vi "Agilent 428X Series Calculated Accuracy Application.vi"(8 "error in (no error)":errorcluster, 9 "Meas. Type (0:Z,Y)":T1(ring), 10 "Temperature (5 C)":dbl=5.0 min=5.0 max=45.0 format="%.2f", 11 "VISA resource name":refnum<visa-resource-name>) -> (0 "error out":errorcluster, 1 "Relative Accuracy":dbl format="%.3f", 2 "Absolute Accuracy":dbl format="%.3f", 3 "VISA resource name out":refnum<visa-resource-name>)   [LabVIEW 2015]
doc: "This application VI is to calulate the absolute and relative accuracy of user specified type measurement, Application VI can calculate \nZ,Y,L,C R,X.G, B, D, Q, Theta, Rp, and Rs absolute and relative accuracy."
uses:
  <instrlib>/Agilent 428X Series/Agilent 428X Series.lvlib
panel:
  # "© Copyright 2005 National Instruments Corporation.  All Rights Reserved."
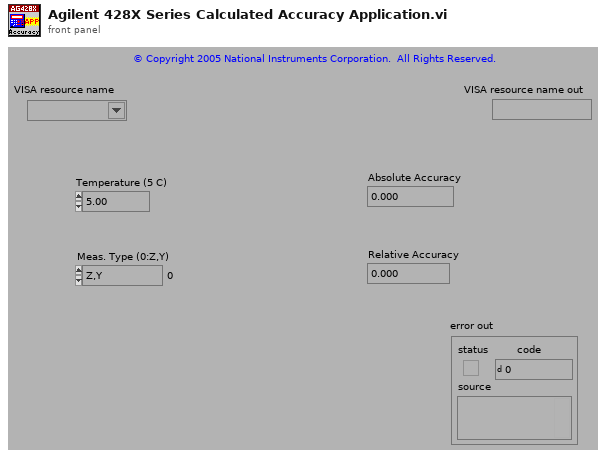
[diagram p1: front panel]
types:
  T1 = enum16{"Z,Y", "L C X B", "R G", "D", "Q", "DEGREE", "G(Cp-G Lp-G)", "Rp", "Rs"}
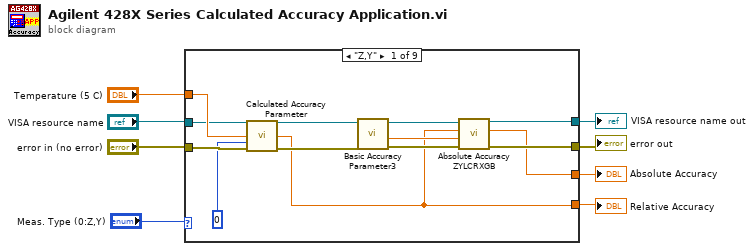
[diagram p0: block diagram]
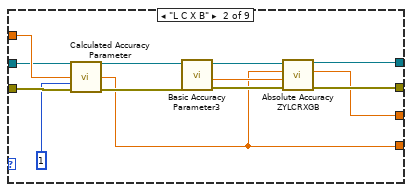
[diagram p2: hidden frame]
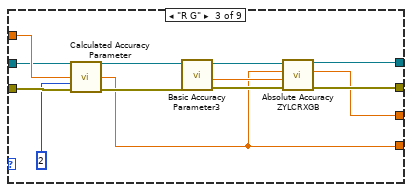
[diagram p3: hidden frame]
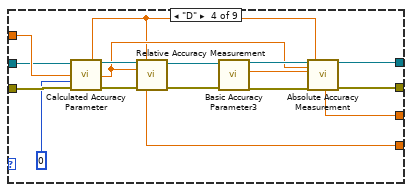
[diagram p4: hidden frame]
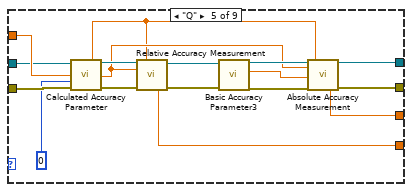
[diagram p5: hidden frame]
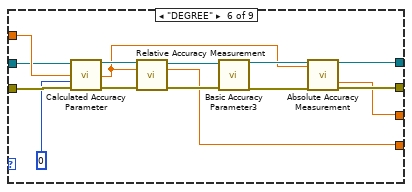
[diagram p6: hidden frame]
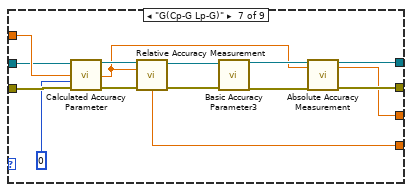
[diagram p7: hidden frame]
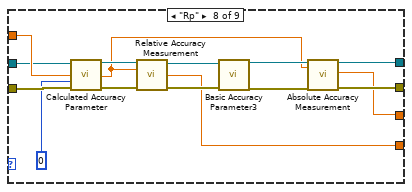
[diagram p8: hidden frame]
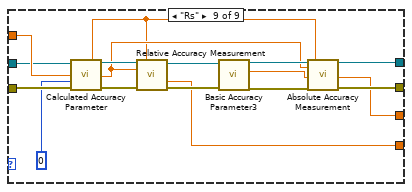
[diagram p9: hidden frame]
diagram:
  n1 = case shown="\"Z,Y\"" "Meas. Type (0:Z,Y)" {
    tunnel: "Temperature (5 C)" -> [w21 w34 w47 w64 w81 w96 w111 w126 w143]
    tunnel: "VISA resource name" -> [w20 w33 w46 w63 w80 w95 w110 w125 w142]
    tunnel: "error in (no error)" -> [w19 w32 w45 w62 w79 w94 w109 w124 w141]
    tunnel: [w13 w26 w39 w49 w68 w82 w97 w112 w127] -> w4
    tunnel: [w11 w24 w37 w58 w75 w90 w105 w120 w137] -> w3
    tunnel: [w10 w23 w36 w57 w74 w89 w104 w119 w136] -> w2
    tunnel: [w9 w22 w35 w52 w67 w84 w98 w113 w130] -> w1
    frame "Z,Y" {
      n2 = call <instrlib>:"Calculated Accuracy Parameter.vi"("VISA resource name"=w20, "Temperature (5 C)"=w21, "Meas. Type (0:Z,Y)"=0, "error in (no error)"=w19) -> ("VISA resource name out"=w18:refnum<visa-resource-name>, "Ae Accuracy"=w13:dbl, "error out"=w17:errorcluster)  [unwired: 8 in, 1 out]
      n3 = call <instrlib>:"Basic Accuracy Parameter3.vi"("error in (no error)"=w17, "VISA resource name"=w18) -> ("error out"=w16:errorcluster, "Acal"=w14:dbl, "VISA resource name out"=w15:refnum<visa-resource-name>)  [unwired: 6 in, 1 out]
      n4 = call <instrlib>:"Absolute Accuracy ZYLCRXGB.vi"("error in (no error)"=w16, "Acal"=w14, "Ae"=w13, "VISA resource name"=w15) -> ("error out"=w10:errorcluster, "Absolute Accuracy"=w9:dbl, "VISA resource name out"=w11:refnum<visa-resource-name>)  [unwired: 5 in]
    }
    frame "L C X B" {
      n5 = call <instrlib>:"Calculated Accuracy Parameter.vi"("VISA resource name"=w33, "Temperature (5 C)"=w34, "Meas. Type (0:Z,Y)"=1, "error in (no error)"=w32) -> ("VISA resource name out"=w31:refnum<visa-resource-name>, "Ae Accuracy"=w26:dbl, "error out"=w30:errorcluster)  [unwired: 8 in, 1 out]
      n6 = call <instrlib>:"Basic Accuracy Parameter3.vi"("error in (no error)"=w30, "VISA resource name"=w31) -> ("error out"=w29:errorcluster, "Acal"=w27:dbl, "VISA resource name out"=w28:refnum<visa-resource-name>)  [unwired: 6 in, 1 out]
      n7 = call <instrlib>:"Absolute Accuracy ZYLCRXGB.vi"("error in (no error)"=w29, "Acal"=w27, "Ae"=w26, "VISA resource name"=w28) -> ("error out"=w23:errorcluster, "Absolute Accuracy"=w22:dbl, "VISA resource name out"=w24:refnum<visa-resource-name>)  [unwired: 5 in]
    }
    frame "R G" {
      n8 = call <instrlib>:"Calculated Accuracy Parameter.vi"("VISA resource name"=w46, "Temperature (5 C)"=w47, "Meas. Type (0:Z,Y)"=2, "error in (no error)"=w45) -> ("VISA resource name out"=w44:refnum<visa-resource-name>, "Ae Accuracy"=w39:dbl, "error out"=w43:errorcluster)  [unwired: 8 in, 1 out]
      n9 = call <instrlib>:"Basic Accuracy Parameter3.vi"("error in (no error)"=w43, "VISA resource name"=w44) -> ("error out"=w42:errorcluster, "Acal"=w40:dbl, "VISA resource name out"=w41:refnum<visa-resource-name>)  [unwired: 6 in, 1 out]
      n10 = call <instrlib>:"Absolute Accuracy ZYLCRXGB.vi"("error in (no error)"=w42, "Acal"=w40, "Ae"=w39, "VISA resource name"=w41) -> ("error out"=w36:errorcluster, "Absolute Accuracy"=w35:dbl, "VISA resource name out"=w37:refnum<visa-resource-name>)  [unwired: 5 in]
    }
    frame "D" {
      n11 = call <instrlib>:"Calculated Accuracy Parameter.vi"("VISA resource name"=w63, "Temperature (5 C)"=w64, "Meas. Type (0:Z,Y)"=0, "error in (no error)"=w62) -> ("Frequency Used"=w48:dbl, "VISA resource name out"=w56:refnum<visa-resource-name>, "Ae Accuracy"=w51:dbl, "error out"=w55:errorcluster)  [unwired: 8 in]
      n12 = call <instrlib>:"Relative Accuracy Measurement.vi"("VISA resource name"=w56, "Frequency (20)"=w48, "Ae Accuracy (0.05)"=w51, "error in (no error)"=w55) -> ("VISA resource name out"=w54:refnum<visa-resource-name>, "D Accuracy"=w49:dbl, "error out"=w53:errorcluster)  [unwired: 4 in, 5 out]
      n13 = call <instrlib>:"Basic Accuracy Parameter3.vi"("error in (no error)"=w53, "VISA resource name"=w54) -> ("error out"=w61:errorcluster, "Radcal"=w50:dbl, "VISA resource name out"=w60:refnum<visa-resource-name>)  [unwired: 6 in, 1 out]
      n14 = call <instrlib>:"Absolute Accuracy Measurement.vi"("VISA resource name"=w60, "Ae Accuracy (0.05)"=w51, "Radcal"=w50, "error in (no error)"=w61, "Frequency (20)"=w48) -> ("D Accuracy"=w52:dbl, "VISA resource name out"=w58:refnum<visa-resource-name>, "error out"=w57:errorcluster)  [unwired: 7 in, 5 out]
    }
    frame "Q" {
      n15 = call <instrlib>:"Calculated Accuracy Parameter.vi"("VISA resource name"=w80, "Temperature (5 C)"=w81, "Meas. Type (0:Z,Y)"=0, "error in (no error)"=w79) -> ("Frequency Used"=w66:dbl, "VISA resource name out"=w73:refnum<visa-resource-name>, "Ae Accuracy"=w69:dbl, "error out"=w72:errorcluster)  [unwired: 8 in]
      n16 = call <instrlib>:"Relative Accuracy Measurement.vi"("VISA resource name"=w73, "Frequency (20)"=w66, "Ae Accuracy (0.05)"=w69, "error in (no error)"=w72) -> ("VISA resource name out"=w71:refnum<visa-resource-name>, "Q Accuracy"=w68:dbl, "error out"=w70:errorcluster)  [unwired: 4 in, 5 out]
      n17 = call <instrlib>:"Basic Accuracy Parameter3.vi"("error in (no error)"=w70, "VISA resource name"=w71) -> ("error out"=w78:errorcluster, "Radcal"=w65:dbl, "VISA resource name out"=w77:refnum<visa-resource-name>)  [unwired: 6 in, 1 out]
      n18 = call <instrlib>:"Absolute Accuracy Measurement.vi"("VISA resource name"=w77, "Ae Accuracy (0.05)"=w69, "Radcal"=w65, "error in (no error)"=w78, "Frequency (20)"=w66) -> ("Q Accuracy"=w67:dbl, "VISA resource name out"=w75:refnum<visa-resource-name>, "error out"=w74:errorcluster)  [unwired: 7 in, 5 out]
    }
    frame "DEGREE" {
      n19 = call <instrlib>:"Calculated Accuracy Parameter.vi"("VISA resource name"=w95, "Temperature (5 C)"=w96, "Meas. Type (0:Z,Y)"=0, "error in (no error)"=w94) -> ("VISA resource name out"=w88:refnum<visa-resource-name>, "Ae Accuracy"=w83:dbl, "error out"=w87:errorcluster)  [unwired: 8 in, 1 out]
      n20 = call <instrlib>:"Relative Accuracy Measurement.vi"("VISA resource name"=w88, "Ae Accuracy (0.05)"=w83, "error in (no error)"=w87) -> ("VISA resource name out"=w86:refnum<visa-resource-name>, "Degree Accuracy"=w82:dbl, "error out"=w85:errorcluster)  [unwired: 5 in, 5 out]
      n21 = call <instrlib>:"Basic Accuracy Parameter3.vi"("error in (no error)"=w85, "VISA resource name"=w86) -> ("error out"=w93:errorcluster, "VISA resource name out"=w92:refnum<visa-resource-name>)  [unwired: 6 in, 2 out]
      n22 = call <instrlib>:"Absolute Accuracy Measurement.vi"("VISA resource name"=w92, "Ae Accuracy (0.05)"=w83, "error in (no error)"=w93) -> ("VISA resource name out"=w90:refnum<visa-resource-name>, "Deg Accuracy"=w84:dbl, "error out"=w89:errorcluster)  [unwired: 9 in, 5 out]
    }
    frame "G(Cp-G Lp-G)" {
      n23 = call <instrlib>:"Calculated Accuracy Parameter.vi"("VISA resource name"=w110, "Temperature (5 C)"=w111, "Meas. Type (0:Z,Y)"=0, "error in (no error)"=w109) -> ("VISA resource name out"=w103:refnum<visa-resource-name>, "Ae Accuracy"=w99:dbl, "error out"=w102:errorcluster)  [unwired: 8 in, 1 out]
      n24 = call <instrlib>:"Relative Accuracy Measurement.vi"("VISA resource name"=w103, "Ae Accuracy (0.05)"=w99, "error in (no error)"=w102) -> ("VISA resource name out"=w101:refnum<visa-resource-name>, "G Accuracy"=w97:dbl, "error out"=w100:errorcluster)  [unwired: 5 in, 5 out]
      n25 = call <instrlib>:"Basic Accuracy Parameter3.vi"("error in (no error)"=w100, "VISA resource name"=w101) -> ("error out"=w108:errorcluster, "VISA resource name out"=w107:refnum<visa-resource-name>)  [unwired: 6 in, 2 out]
      n26 = call <instrlib>:"Absolute Accuracy Measurement.vi"("VISA resource name"=w107, "Ae Accuracy (0.05)"=w99, "error in (no error)"=w108) -> ("VISA resource name out"=w105:refnum<visa-resource-name>, "G Accuracy"=w98:dbl, "error out"=w104:errorcluster)  [unwired: 9 in, 5 out]
    }
    frame "Rp" {
      n27 = call <instrlib>:"Calculated Accuracy Parameter.vi"("VISA resource name"=w125, "Temperature (5 C)"=w126, "Meas. Type (0:Z,Y)"=0, "error in (no error)"=w124) -> ("VISA resource name out"=w118:refnum<visa-resource-name>, "Ae Accuracy"=w114:dbl, "error out"=w117:errorcluster)  [unwired: 8 in, 1 out]
      n28 = call <instrlib>:"Relative Accuracy Measurement.vi"("VISA resource name"=w118, "Ae Accuracy (0.05)"=w114, "error in (no error)"=w117) -> ("VISA resource name out"=w116:refnum<visa-resource-name>, "Rp Accuracy"=w112:dbl, "error out"=w115:errorcluster)  [unwired: 5 in, 5 out]
      n29 = call <instrlib>:"Basic Accuracy Parameter3.vi"("error in (no error)"=w115, "VISA resource name"=w116) -> ("error out"=w123:errorcluster, "VISA resource name out"=w122:refnum<visa-resource-name>)  [unwired: 6 in, 2 out]
      n30 = call <instrlib>:"Absolute Accuracy Measurement.vi"("VISA resource name"=w122, "Ae Accuracy (0.05)"=w114, "error in (no error)"=w123) -> ("VISA resource name out"=w120:refnum<visa-resource-name>, "Rp Accuracy"=w113:dbl, "error out"=w119:errorcluster)  [unwired: 9 in, 5 out]
    }
    frame "Rs" {
      n31 = call <instrlib>:"Calculated Accuracy Parameter.vi"("VISA resource name"=w142, "Temperature (5 C)"=w143, "Meas. Type (0:Z,Y)"=0, "error in (no error)"=w141) -> ("Frequency Used"=w129:dbl, "VISA resource name out"=w135:refnum<visa-resource-name>, "Ae Accuracy"=w131:dbl, "error out"=w134:errorcluster)  [unwired: 8 in]
      n32 = call <instrlib>:"Relative Accuracy Measurement.vi"("VISA resource name"=w135, "Frequency (20)"=w129, "Ae Accuracy (0.05)"=w131, "error in (no error)"=w134) -> ("VISA resource name out"=w133:refnum<visa-resource-name>, "Rs Accuracy"=w127:dbl, "error out"=w132:errorcluster)  [unwired: 4 in, 5 out]
      n33 = call <instrlib>:"Basic Accuracy Parameter3.vi"("error in (no error)"=w132, "VISA resource name"=w133) -> ("error out"=w140:errorcluster, "Radcal"=w128:dbl, "VISA resource name out"=w139:refnum<visa-resource-name>)  [unwired: 6 in, 1 out]
      n34 = call <instrlib>:"Absolute Accuracy Measurement.vi"("VISA resource name"=w139, "Ae Accuracy (0.05)"=w131, "Radcal"=w128, "error in (no error)"=w140, "Frequency (20)"=w129) -> ("VISA resource name out"=w137:refnum<visa-resource-name>, "Rs Accuracy"=w130:dbl, "error out"=w136:errorcluster)  [unwired: 7 in, 5 out]
    }
  }
  "error out" <- w2
  "VISA resource name out" <- w3
  "Absolute Accuracy" <- w1
  "Relative Accuracy" <- w4
